vi "Test API if the vi pane control refs are basic types.vi"(8 "error in (no error)":errorcluster, 11 "TestCase in":refnum<class "Test Scripting API.lvclass">) -> (0 "error out":errorcluster, 3 "TestCase out":refnum<class "Test Scripting API.lvclass">)   [LabVIEW 2020, in "Test Scripting API.lvclass"]
uses:
  Test Scripting API.lvclass
  <vilib>/Utility/Data Type/Type Definitions/Data Type.ctl
  VI UUT.vi
  Scripting Playground/Scripting/DQMH_API.lvlib
  <vilib>/Utility/Data Type/NI_Data Type.lvlib
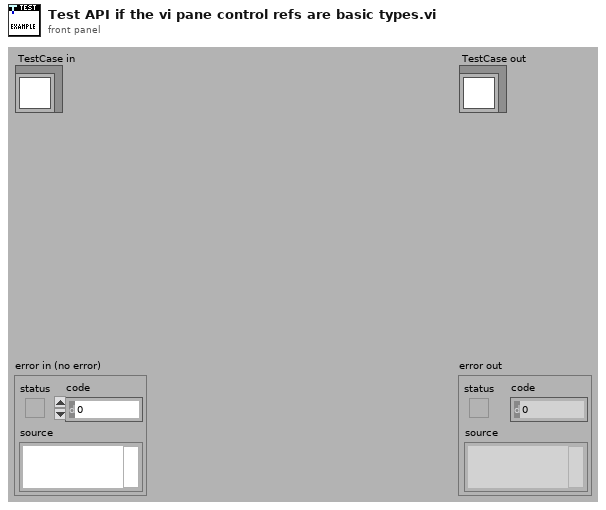
[diagram p1: front panel]
types:
  T1 = typedef "NI_Data Type.lvlib/Data Type.ctl" = enum8{"Invalid Type", "Void", "I8", "I16", "I32", "I64", "U8", "U16", "U32", "U64", "Single Float", "Double Float", "Extended Float", "Single Complex", "Double Complex", "Extended Complex", "Enum U8", "Enum U16", "Enum U32", "Enum U64", "Single Float With Unit", "Double Float With Unit", "Extended Float With Unit", "Single Complex with Unit", "Double Complex with Unit", "Extended Complex with Unit", "Boolean", "String", "Path", "Picture", "Tag", "Array", "Cluster", "Variant", "LV Variant", "Waveform", "Timestamp", "Digital Waveform", "Digital Data", "ExpressData", "Refnum", "External Data", "VI", "Poly VI", "LabVIEW Class Instance", "Fixed Point", "Set Collection", "Map Collection"}
  T2 = typedef "DQMH_API.lvlib/Controls Refs and Type--cluster.ctl" = cluster{"Ctrls Refs ":refnum<vi>[], "Ctrls Types":T1[], "Names":string[]}
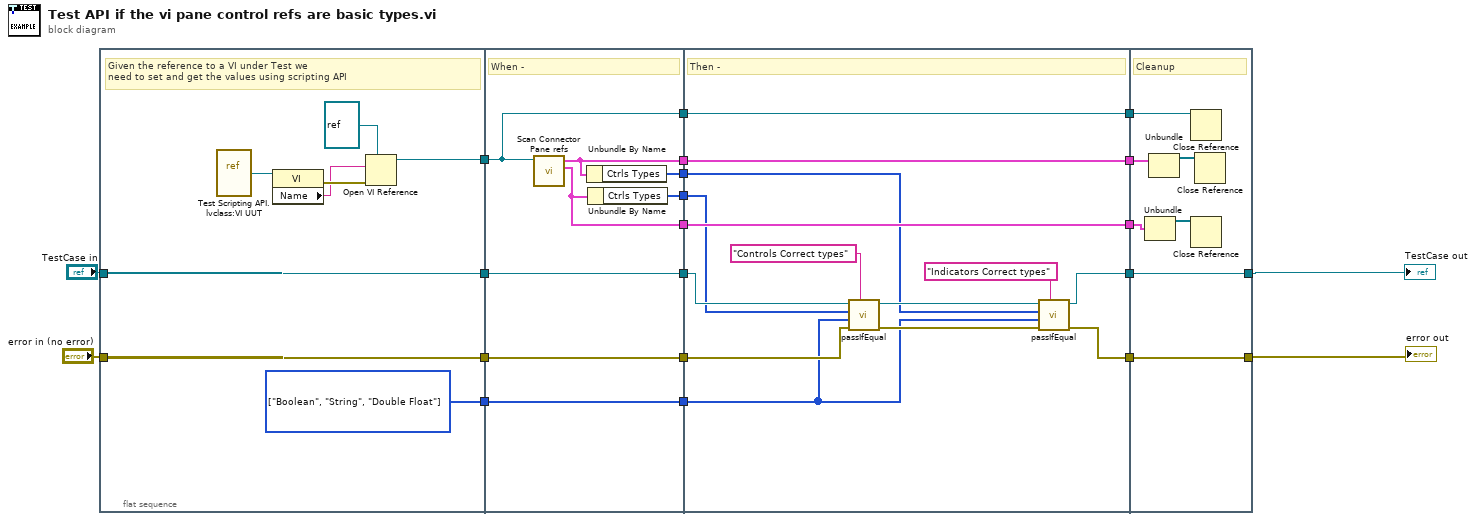
[diagram p0: block diagram]
diagram:
  n1 = flat-sequence {
    tunnel: "error in (no error)" -> [w28]
    tunnel: "TestCase in" -> [w29]
    tunnel: [w29] -> w21
    tunnel: [w28] -> w20
    tunnel: [w23] -> w10
    tunnel: [w22] -> w1
    tunnel: [w37] -> w19
    tunnel: [w36] -> w18
    tunnel: w21 -> [w37]
    tunnel: w20 -> [w36]
    tunnel: [w33] -> w11
    tunnel: w10 -> [w35]
    tunnel: [w35] -> w9
    tunnel: [w34] -> w5
    tunnel: [w32] -> w4
    tunnel: [w31] -> w3
    tunnel: [w30] -> w2
    tunnel: w1 -> [w30]
    tunnel: [w46] -> w17
    tunnel: [w48] -> w16
    tunnel: w19 -> [w51]
    tunnel: w18 -> [w50]
    tunnel: w11 -> [w44]
    tunnel: w9 -> [w45]
    tunnel: [w45] -> w8
    tunnel: [w44] -> w7
    tunnel: [w43] -> w6
    tunnel: w5 -> [w43]
    tunnel: w4 -> [w41]
    tunnel: w3 -> [w42]
    tunnel: w2 -> [w40]
    tunnel: [w57] -> w13
    tunnel: [w58] -> w12
    tunnel: w17 -> [w58]
    tunnel: w16 -> [w57]
    tunnel: w8 -> [w56]
    tunnel: w7 -> [w54]
    tunnel: w6 -> [w55]
    frame #0 {
      w22 = T1[] [enum."Boolean", enum."String", enum."Double Float"] items=["Invalid Type", "Void", "I8", "I16", "I32", "I64", "U8", "U16", "U32", "U64", "Single Float", "Double Float", "Extended Float", "Single Complex", "Double Complex", "Extended Complex", "Enum U8", "Enum U16", "Enum U32", "Enum U64", "Single Float With Unit", "Double Float With Unit", "Extended Float With Unit", "Single Complex with Unit", "Double Complex with Unit", "Extended Complex with Unit", "Boolean", "String", "Path", "Picture", "Tag", "Array", "Cluster", "Variant", "LV Variant", "Waveform", "Timestamp", "Digital Waveform", "Digital Data", "ExpressData", "Refnum", "External Data", "VI", "Poly VI", "LabVIEW Class Instance", "Fixed Point", "Set Collection", "Map Collection"] ("Ctrls Types")
      # "Given the reference to a VI under Test we\nneed to set and get the values using scripting API"
      n2 = vi-ref "Test Scripting API.lvclass:VI UUT.vi"() -> (w26:refnum<vi>)
      n3 = property class="VI"(reference=w26) -> (error out=w27:errorcluster, "Name"=w25:string)  [unwired: 1 in, 1 out]
      n4 = Open VI Reference(type specifier VI Refnum (for type only)=refnum<vi> refnum, vi path=w25, error in (no error)=w27) -> (vi reference=w23:refnum<vi>)  [unwired: 3 in, 1 out]
    }
    frame #1 {
      # "When -"
      n5 = call "Scan Connector Pane refs.vi"("VI in"=w35) -> ("Controls"=w34:T2, "Indicators"=w33:T2)  [unwired: 9 in]
      n6 = Unbundle By Name(w33) -> ("Ctrls Types"=w32:T1[])
      n7 = Unbundle By Name(w34) -> ("Ctrls Types"=w31:T1[])
    }
    frame #2 {
      # "Then -"
      n8 = call-dynamic "passIfEqual.vi"("custom report message (\"\")"="Controls Correct types" ("custom report message (\"\")"), "error in (no error)"=w50, "y"=w40, "x"=w42, "TestCase in"=w51) -> ("error out"=w49:errorcluster, "TestCase out"=w47:refnum<class "Test Scripting API.lvclass">)  [unwired: 5 in]
      n9 = call-dynamic "passIfEqual.vi"("custom report message (\"\")"="Indicators Correct types" ("custom report message (\"\")"), "error in (no error)"=w49, "y"=w40, "x"=w41, "TestCase in"=w47) -> ("error out"=w48:errorcluster, "TestCase out"=w46:refnum<class "Test Scripting API.lvclass">)  [unwired: 5 in]
    }
    frame #3 {
      # "Cleanup"
      n10 = Unbundle(w55) -> ("Ctrls Refs"=w52:refnum<vi>[])  [unwired: 2 out]
      n11 = Unbundle(w54) -> ("Ctrls Refs"=w53:refnum<vi>[])  [unwired: 2 out]
      n12 = Close Reference(reference=w56) -> ()  [unwired: 1 in, 1 out]
      n13 = Close Reference(reference=w52) -> ()  [unwired: 1 in, 1 out]
      n14 = Close Reference(reference=w53) -> ()  [unwired: 1 in, 1 out]
    }
  }
  "error out" <- w13
  "TestCase out" <- w12
